vi "CPU Log.vi"(10 "Total CPU %":dbl format="%#_13g") -> ()   [LabVIEW 2019]
uses:
  <vilib>/Utility/file.llb/Write Delimited Spreadsheet (string).vi
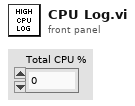
[diagram p1: front panel]
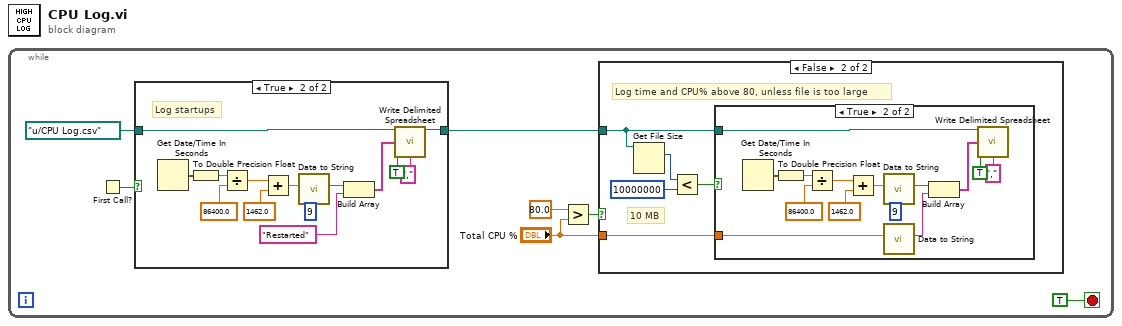
[diagram p0: block diagram]
diagram:
  n1 = while {
    stop <- TRUE stop-if-true
    n2 = First Call?() -> (First Call?: T/F=w6:bool)
    n3 = case shown="True" w6 {
      tunnel: path "u:/CPU Log.csv" ("Fuel Log Path") -> [w27 w32]
      tunnel: [w27 w31] -> w4
      frame False {
      }
      frame True {
        # "Log startups"
        n4 = Get Date/Time In Seconds() -> (seconds since 1Jan1904=w36:timestamp)
        n5 = To Double Precision Float(number=w36) -> (double precision float=w35:dbl)
        n6 = Divide(x=w35, y=86400.0) -> (x/y=w39:dbl)
        n7 = Add(x=w39, y=1462.0) -> (x+y=w40:dbl)
        n8 = call "Data to String.vi"("Precision (2)"=i16 9, "Data"=w40) -> ("String Data"=w34:string)  [unwired: 9 in]
        n9 = Build Array(w34, "Restarted") -> (w28:string[])
        n10 = call-poly <vilib>:"Write Delimited Spreadsheet.vi"("file path (dialog if empty)"=w32, "1D data"=w28, "append to file? (new file:F)"=TRUE, "delimiter (\\t)"="," ("delimiter (\\t)")) -> ("new file path (Not A Path if cancelled)"=w31:path)  [unwired: 10 in, 1 out]
      }
    }
    n11 = Greater?(x=80.0, y="Total CPU %") -> (0:w2:bool)
    n12 = case shown="False" w2 {
      tunnel: w4 -> [_ w11]
      tunnel: "Total CPU %" -> [_ w12]
      frame True {
      }
      frame False {
        # "Log time and CPU% above 80, unless file is too large"
        # "10 MB"
        n13 = Get File Size(file=w11) -> (size (in bytes)=w10:i64)  [unwired: 1 in, 2 out]
        n14 = Less?(x=w10, y=i64 10000000) -> (x < y?=w8:bool)
        n15 = case shown="True" w8 {
          tunnel: w11 -> [_ w18]
          tunnel: w12 -> [_ w17]
          frame False {
          }
          frame True {
            n16 = Get Date/Time In Seconds() -> (seconds since 1Jan1904=w24:timestamp)
            n17 = To Double Precision Float(number=w24) -> (double precision float=w25:dbl)
            n18 = Divide(x=w25, y=86400.0) -> (x/y=w21:dbl)
            n19 = Add(x=w21, y=1462.0) -> (x+y=w20:dbl)
            n20 = call "Data to String.vi"("Precision (2)"=i16 9, "Data"=w20) -> ("String Data"=w26:string)  [unwired: 9 in]
            n21 = call "Data to String.vi"("Data"=w17) -> ("String Data"=w16:string)  [unwired: 10 in]
            n22 = Build Array(w26, w16) -> (w13:string[])
            n23 = call-poly <vilib>:"Write Delimited Spreadsheet.vi"("file path (dialog if empty)"=w18, "1D data"=w13, "append to file? (new file:F)"=TRUE, "delimiter (\\t)"="," ("delimiter (\\t)")) -> ()  [unwired: 10 in, 2 out]
          }
        }
      }
    }
  }
